vi "GUI Main.vi"() -> ()   [LabVIEW 2014]
panel:
  out "Heater Status":bool
  in  "Boolean":bool
  out "Main Power":bool
  out "Temp Diff ( target - actual )":string
  out "Target":string
  in  "OK Button":bool
  in  "target input":dbl
  out "Temperat3":string
  out "Water Temperature":string
  out "Thermometer":dbl(slide) scale=0.0..100.0
  out "Waveform Chart":dbl(graph)
  out "Error Out":errorcluster
  in  "Stop Button":bool
  out "GUI status":string="Hello"
  # "Water Temperature Control"
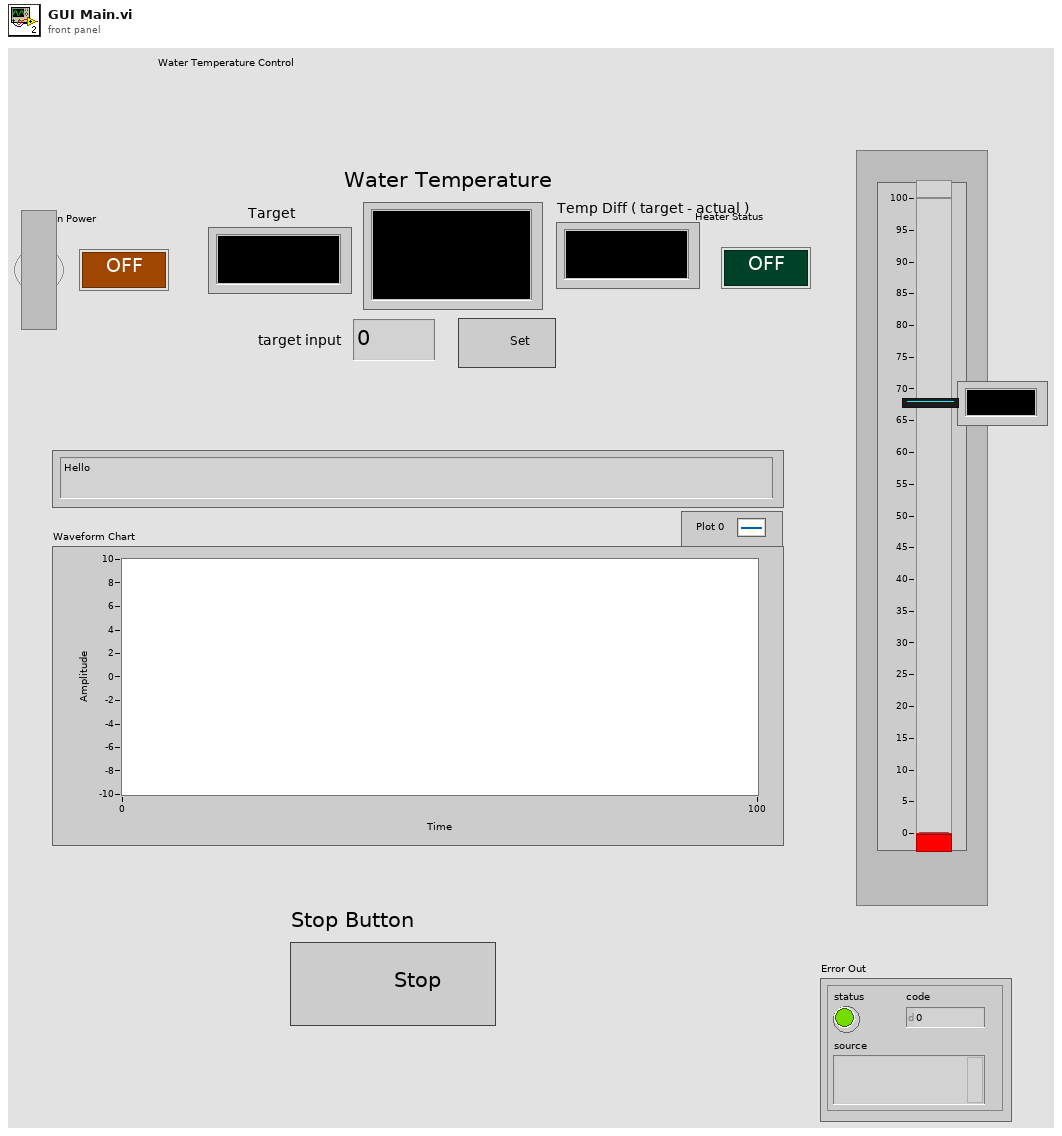
[diagram p1: front panel]
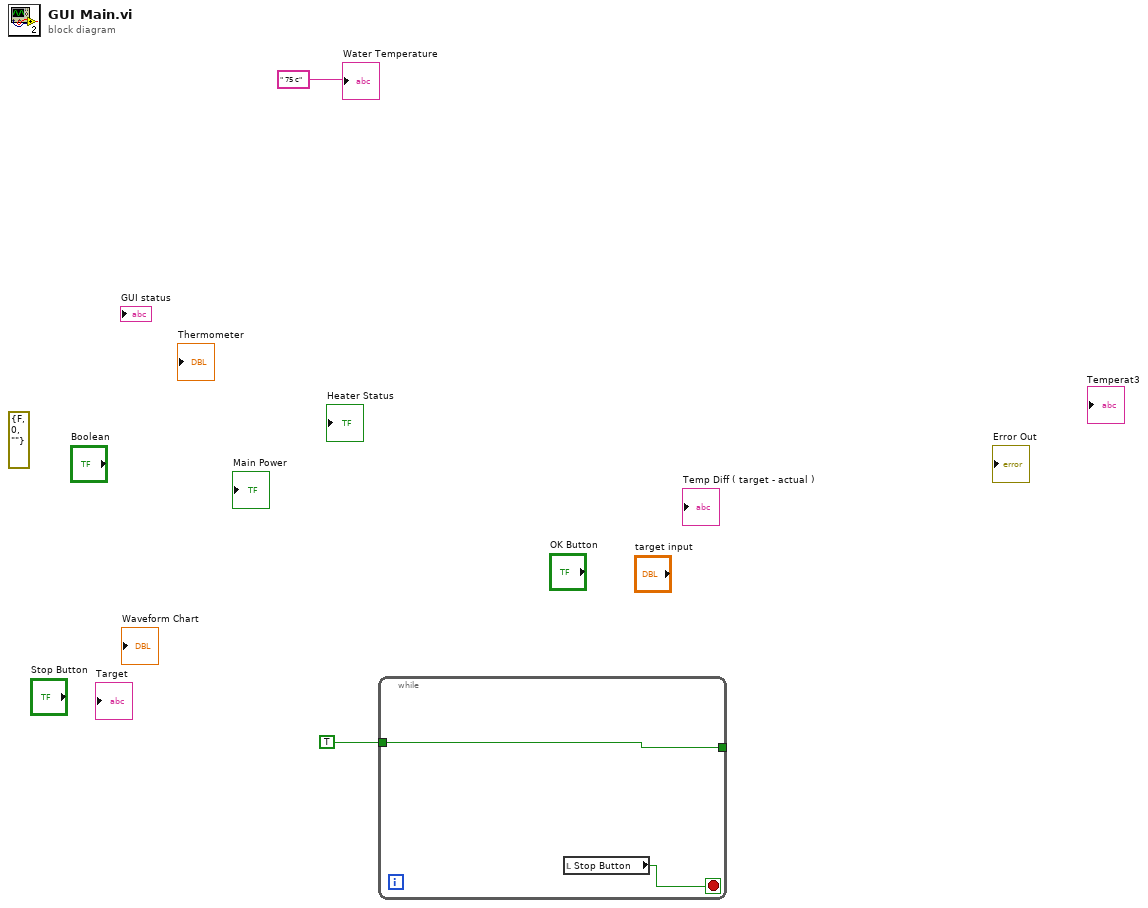
[diagram p0: block diagram]
diagram:
  (unwired) errorcluster {"status"=FALSE, "code"=0, "source"=""} ("Error In")
  n1 = while {
    tunnel: [w3] -> _
    tunnel: TRUE -> [w3]
    stop <- w4 stop-if-true
    n2 = local read "Stop Button"() -> (w4:bool)
  }
  "Water Temperature" <- " 75 c"
